vi "Chord to Center.vi"(11 "Tag points":T1) -> (1 "output circle info":T2, 2 "T2 endPt":cluster{dbl, dbl}, 3 "T1 endPt":cluster{dbl, dbl}, 4 "angle T1 to T2":dbl)   [LabVIEW 2023]
uses:
  <vilib>/vision/NI_Vision_Development_Module.lvlib
panel:
  in  "stroke length":dbl=10.0 format="%#_13g"
  out "delta angle":dbl
  out "length of chord":dbl
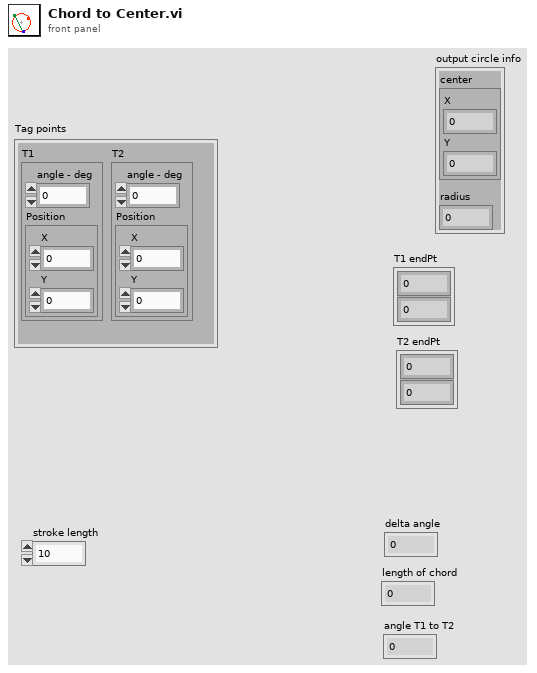
[diagram p1: front panel]
types:
  T1 = cluster{"T1":cluster{"angle - deg":dbl, "Position":cluster{"X":dbl, "Y":dbl}}, "T2":cluster{"angle - deg":dbl, "Position":cluster{"X":dbl, "Y":dbl}}}
  T2 = cluster{"center":cluster{"X":sgl, "Y":sgl}, "radius":sgl}
  T3 = cluster{"angle - deg":dbl, "Position":cluster{"X":dbl, "Y":dbl}}
  T4 = cluster{"Position":cluster{"X":dbl, "Y":dbl}, cluster{dbl, dbl}}
  T5 = cluster{"Intersection Point":cluster{"X":sgl, "Y":sgl}, sgl}
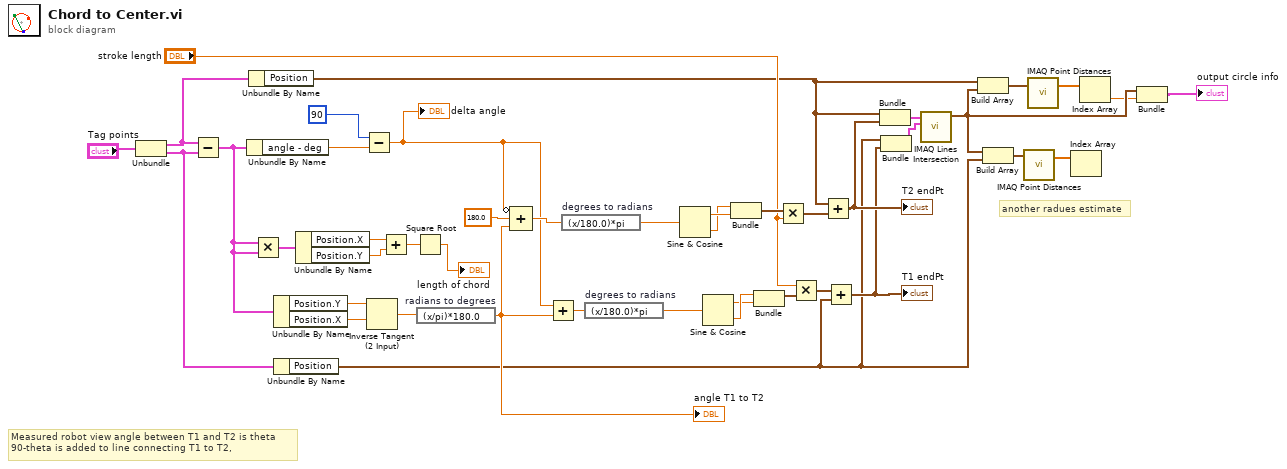
[diagram p0: block diagram]
diagram:
  # "another radues estimate"
  # "Measured robot view angle between T1 and T2 is theta\n90-theta is added to line connecting T1 to T2,"
  n1 = Unbundle("Tag points") -> ("T1"=w2:T3, "T2"=w1:T3)
  n2 = Subtract(x=w2, y=w1) -> (x-y=w31:T3)
  n3 = Unbundle By Name(w31) -> ("angle - deg"=w7:dbl)
  n4 = Unbundle By Name(w2) -> ("Position"=w13:cluster{"X":dbl, "Y":dbl})
  n5 = Multiply(x=w31, y=w31) -> (x*y=w27:T3)
  n6 = Unbundle By Name(w31) -> ("Position.Y"=w32:dbl, "Position.X"=w33:dbl)
  n7 = Unbundle By Name(w1) -> ("Position"=w11:cluster{"X":dbl, "Y":dbl})
  n8 = Unbundle By Name(w27) -> ("Position.X"=w28:dbl, "Position.Y"=w29:dbl)
  n9 = Subtract(x=90, y=w7) -> (x-y=w18:dbl)
  "delta angle" <- w18
  n10 = Inverse Tangent (2 Input)(1:w33, 2:w32) -> (0:w34:dbl)
  n11 = Add(x=w28, y=w29) -> (x+y=w30:dbl)
  n12 = Square Root(x=w30) -> (sqrt(x)=→"length of chord":dbl)
  n13 = expression code="(x/pi)*180.0" "radians to degrees"(w34) -> (w42:dbl)
  "angle T1 to T2" <- w42
  n14 = Compound Arithmetic op=ADD(invert w18, 180.0 ("x"), w42) -> (w22:dbl)
  n15 = Add(x=w18, y=w42) -> (x+y=w40:dbl)
  n16 = expression code="(x/180.0)*pi" "degrees to radians"(w22) -> (w23:dbl)
  n17 = expression code="(x/180.0)*pi" "degrees to radians"(w40) -> (w41:dbl)
  n18 = Sine & Cosine(0:w23) -> (1:w25:dbl, 2:w24:dbl)
  n19 = Sine & Cosine(0:w41) -> (1:w35:dbl, 2:w36:dbl)
  n20 = Bundle(w24, w25) -> (w21:cluster{dbl, dbl})  [unwired: 1 in]
  n21 = Bundle(w36, w35) -> (w37:cluster{dbl, dbl})  [unwired: 1 in]
  n22 = Multiply(x=w21, y="stroke length") -> (x*y=w19:cluster{dbl, dbl})
  n23 = Multiply(x="stroke length", y=w37) -> (x*y=w39:cluster{dbl, dbl})
  n24 = Add(x=w13, y=w19) -> (x+y=w17:cluster{dbl, dbl})
  "T2 endPt" <- w17
  n25 = Add(x=w39, y=w11) -> (x+y=w15:cluster{dbl, dbl})
  "T1 endPt" <- w15
  n26 = Bundle("Position"=w13, w17) -> (w16:T4)  [unwired: 1 in]
  n27 = Bundle("Position"=w11, w15) -> (w14:T4)  [unwired: 1 in]
  n28 = call "IMAQ Lines Intersection"("Line 2"=w14, "Line 1"=w16) -> ("Intersection Point"=w6:cluster{"X":sgl, "Y":sgl})  [unwired: 7 in, 2 out]
  n29 = Build Array(w13, w6) -> (w12:cluster{"X":dbl, "Y":dbl}[])
  n30 = Build Array(w6, w11) -> (w10:cluster{"X":dbl, "Y":dbl}[])
  n31 = call "IMAQ Point Distances"("Points"=w10) -> ("Distances"=w8:sgl[])  [unwired: 4 in, 1 out]
  n32 = call "IMAQ Point Distances"("Points"=w12) -> ("Distances"=w9:sgl[])  [unwired: 4 in, 1 out]
  n33 = Index Array(array=w8) -> ()  [unwired: 1 in, 1 out]
  n34 = Index Array(array=w9) -> (element=w5:sgl)  [unwired: 1 in]
  n35 = Bundle("Intersection Point"=w6, w5) -> (→"output circle info":T5)  [unwired: 1 in]
